vi "获取质控状态.vi"(8 "error in (no error)":errorcluster caption="错误输入（无错误）", 11 "参数":enum16{"氨氮", "总磷", "总氮", "CODMn", "CODcr"}(ring)) -> (0 "error out":errorcluster caption="错误输出", 3 "仪器状态":T1(ring))   [LabVIEW 2016, in "质控单元.lvlib"]
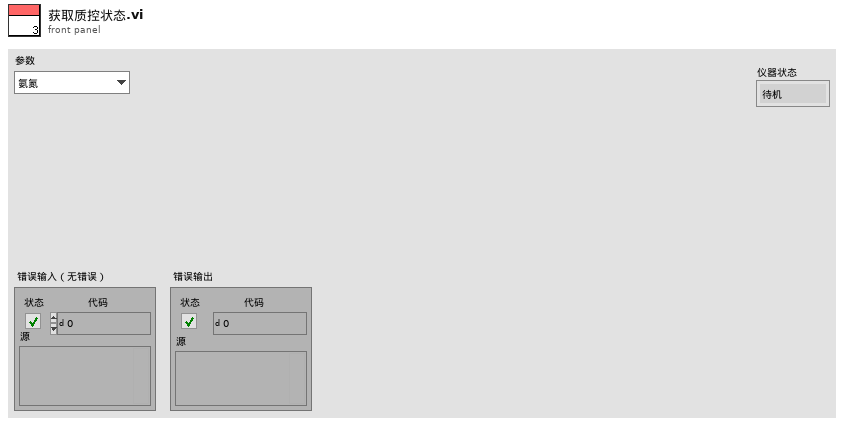
[diagram p1: front panel]
types:
  T1 = enum16{"待机", "润洗中", "进样中", "加标中", "排液中", "搅拌中", "进样超时报警"}
  T2 = cluster{"氨氮":u8, "总磷":u8, "总氮":u8, "CODMn":u8, "CODCr":u8}
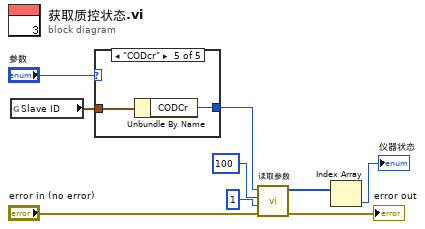
[diagram p0: block diagram]
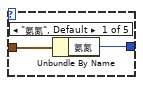
[diagram p2: hidden frame]
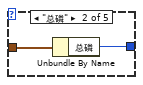
[diagram p3: hidden frame]
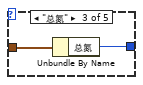
[diagram p4: hidden frame]
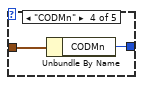
[diagram p5: hidden frame]
diagram:
  n1 = global read "断电保存全局.vi" "Slave ID"() -> (w3:T2)
  n2 = case shown="\"CODcr\"" "参数" {
    tunnel: w3 -> [w11 w13 w15 w17 w19]
    tunnel: [w10 w12 w14 w16 w18] -> w1
    frame "氨氮", Default {
      n3 = Unbundle By Name(w11) -> ("氨氮"=w10:u8)
    }
    frame "总磷" {
      n4 = Unbundle By Name(w13) -> ("总磷"=w12:u8)
    }
    frame "总氮" {
      n5 = Unbundle By Name(w15) -> ("总氮"=w14:u8)
    }
    frame "CODMn" {
      n6 = Unbundle By Name(w17) -> ("CODMn"=w16:u8)
    }
    frame "CODcr" {
      n7 = Unbundle By Name(w19) -> ("CODCr"=w18:u8)
    }
  }
  n8 = call "读取参数.vi"("Slave ID"=w1, "starting address"=u16 100, "quantity"=u16 1, "Error in"="error in (no error)") -> ("values"=w5:u16[], "error out"=→"error out":errorcluster)  [unwired: 5 in]
  n9 = Index Array(array=w5) -> (element=→"仪器状态":u16)  [unwired: 1 in]
